vi "getProjectionRes.vi"() -> (1 "projBounds":T1, 2 "YRes":i32, 3 "XRes":i32)   [LabVIEW 2017]
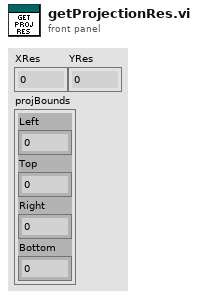
[diagram p1: front panel]
types:
  T1 = cluster{"Left":i32, "Top":i32, "Right":i32, "Bottom":i32}
  T2 = typedef "LVAllMonitorsDisplayTypeDef.ctl" = cluster{"Bounds":cluster{"Left":i16, "Top":i16, "Right":i16, "Bottom":i16}, "Depth":i16}[]
  T3 = cluster{"Bounds":cluster{"Left":i16, "Top":i16, "Right":i16, "Bottom":i16}, "Depth":i16}
  T4 = cluster{"Left":i16, "Top":i16, "Right":i16, "Bottom":i16}
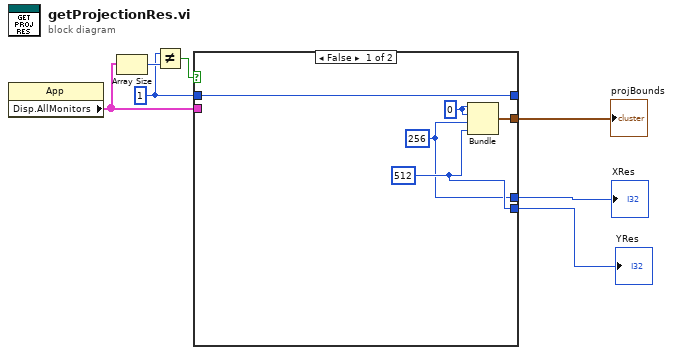
[diagram p0: block diagram]
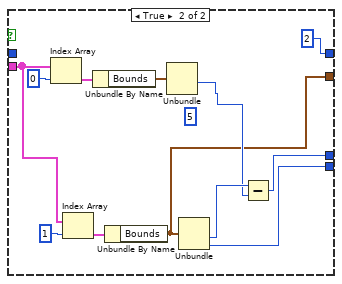
[diagram p2: hidden frame]
diagram:
  w5 = 1 ("x")
  n1 = property class="App"() -> ("Disp.AllMonitors"=w4:T2)  [unwired: 2 in, 2 out]
  n2 = Array Size(array=w4) -> (size(s)=w7:i32)
  n3 = Not Equal?(x=w5, y=w7) -> (x != y?=w6:bool)
  n4 = case shown="False" w6 {
    tunnel: [w12 u16 2 ("Front Panel Window:Monitor")] -> _
    tunnel: w5 -> [w12 _]
    tunnel: w4 -> [_ w19]
    tunnel: [w10 w13] -> w1
    tunnel: [w9 w17] -> w2
    tunnel: [w8 w14] -> w3
    frame False {
      w9 = 512
      w8 = 256
      w11 = 0
      n5 = Bundle(w11, w11, w8, w9) -> (w10:cluster{i32, i32, i32, i32})  [unwired: 1 in]
    }
    frame True {
      (unwired) 5
      n6 = Index Array(array=w19, index=0) -> (element=w23:T3)
      n7 = Index Array(array=w19, index=1) -> (element=w18:T3)
      n8 = Unbundle By Name(w23) -> ("Bounds"=w21:T4)
      n9 = Unbundle By Name(w18) -> ("Bounds"=w13:T4)
      n10 = Unbundle(w21) -> ("Right"=w15:i16)  [unwired: 3 out]
      n11 = Unbundle(w13) -> ("Right"=w16:i16, "Bottom"=w17:i16)  [unwired: 2 out]
      n12 = Subtract(x=w16, y=w15) -> (x-y=w14:i16)
    }
  }
  "XRes" <- w3
  "YRes" <- w2
  "projBounds" <- w1
